vi "Radial_Average_Cleanup.vi"(2 "Radial Resolution":dbl, 3 "Averages":dbl[](array[numeric])) -> (0 "Radius":dbl[](array[numeric]), 1 "Averages":dbl[](array[numeric]))   [LabVIEW 2010]
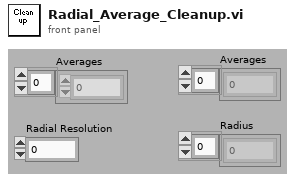
[diagram p1: front panel]
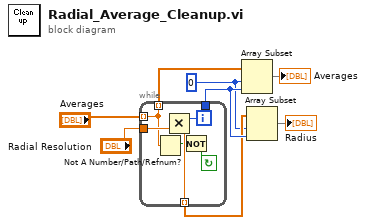
[diagram p0: block diagram]
diagram:
  w1 = 0 ("Array Index")
  n1 = while {
    tunnel: [w11] -> w2 mode=indexing
    tunnel: "Radial Resolution" -> [w12]
    tunnel: [w13] -> w6
    tunnel: "Averages" -> [w9] mode=indexing
    tunnel: [w9] -> w8 mode=indexing
    i -> [w13]
    stop <- w14 continue-if-true
    n2 = Not A Number/Path/Refnum?(number/path/refnum=w9) -> (NaN/Path/Refnum?=w10:bool)
    n3 = Multiply(x=w13, y=w12) -> (x*y=w11:dbl)
    n4 = Not(x=w10) -> (.not. x?=w14:bool)
  }
  n5 = Array Subset(array=w8, index=w1, length=w6) -> (→"Averages":dbl[])
  n6 = Array Subset(array=w2, index=w1, length=w6) -> (→"Radius":dbl[])
